vi "Mem2Num.vi"(8 "Loop":u32=8, 9 "Reset":bool, 11 "Data In":bool) -> (3 "Mem":u8 format="%x")   [LabVIEW 2012]
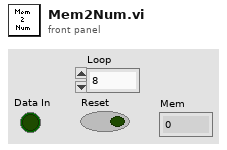
[diagram p1: front panel]
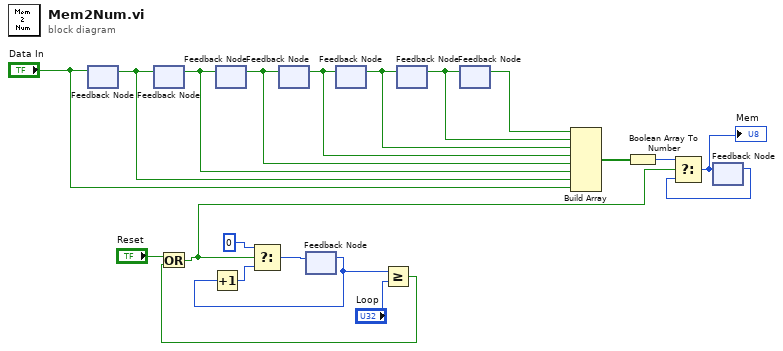
[diagram p0: block diagram]
diagram:
  n1 = feedback-in #1("Data In") -> ()
  n2 = feedback #1() -> (w14:bool)  [unwired: 1 in]
  n3 = feedback #2() -> (w15:bool)  [unwired: 1 in]
  n4 = feedback-in #2(w14) -> ()
  n5 = feedback #3() -> (w16:bool)  [unwired: 1 in]
  n6 = feedback-in #3(w15) -> ()
  n7 = feedback #4() -> (w17:bool)  [unwired: 1 in]
  n8 = feedback-in #4(w16) -> ()
  n9 = feedback #5() -> (w8:u32)  [unwired: 1 in]
  n10 = Increment(x=w8) -> (x+1=w9:u32)
  n11 = feedback #6() -> (w18:bool)  [unwired: 1 in]
  n12 = feedback-in #6(w17) -> ()
  n13 = Greater Or Equal?(x=w8, y="Loop") -> (x >= y?=w6:bool)
  n14 = Or(x="Reset", y=w6) -> (x .or. y?=w1:bool)
  n15 = Select(t=u32 0, s=w1, f=w9) -> (s? t:f=w10:u32)
  n16 = feedback-in #5(w10) -> ()
  n17 = feedback #7() -> (w19:bool)  [unwired: 1 in]
  n18 = feedback-in #7(w18) -> ()
  n19 = feedback #8() -> (w20:bool)  [unwired: 1 in]
  n20 = feedback-in #8(w19) -> ()
  n21 = Build Array(w20, w19, w18, w17, w16, w15, w14, "Data In") -> (w12:bool[])
  n22 = Boolean Array To Number(Boolean array=w12) -> (number=w4:u32)
  n23 = feedback #9() -> (w2:u32)  [unwired: 1 in]
  n24 = Select(t=w4, s=w1, f=w2) -> (s? t:f=w3:u32)
  "Mem" <- w3
  n25 = feedback-in #9(w3) -> ()
